vi "CSM Module Type.vi"(8 "Error in":errorcluster caption="error in (no error)", 11 "CSM Basic Refs":T2) -> (0 "error out":errorcluster, 2 "CSMType":T1, 3 "CSM Basic Refs (dup)":T2)   [LabVIEW 2017, in "CSM-Helper Utility.lvlib"]
doc: "### CSM Module Type.vi\n\n-- <b>Controls</b> --\n- <b>CSM Basic Refs</b>:\n\n-- <b>Indicators</b> --\n- <b>CSM Basic Refs (dup)</b>:"
uses:
  CSM-Helper Utility.lvlib
  CSM Basic Refs.ctl
  CSM Module Type.ctl
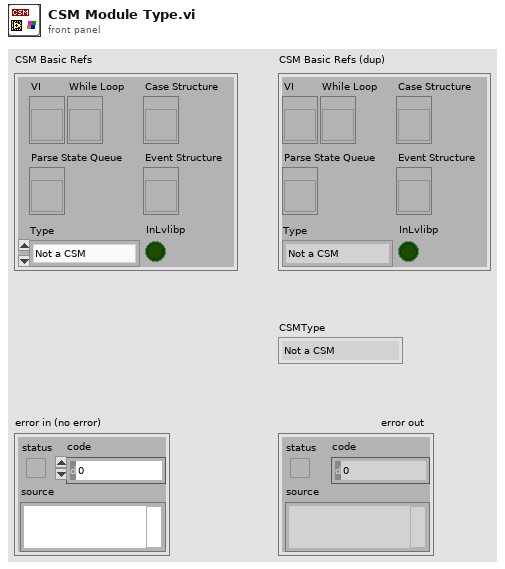
[diagram p1: front panel]
types:
  T1 = typedef "CSM-Helper Utility.lvlib/CSM Module Type.ctl" = enum16{"Not a CSM", "JKISM", "CSM"}
  T2 = typedef "CSM-Helper Utility.lvlib/CSM Basic Refs.ctl" = cluster{"VI":refnum<vi>, "While Loop":refnum<vi>, "Case Structure":refnum<vi>, "Parse State Queue":refnum<vi>, "Event Structure":refnum<vi>, "Type":T1, "InLvlibp":bool}
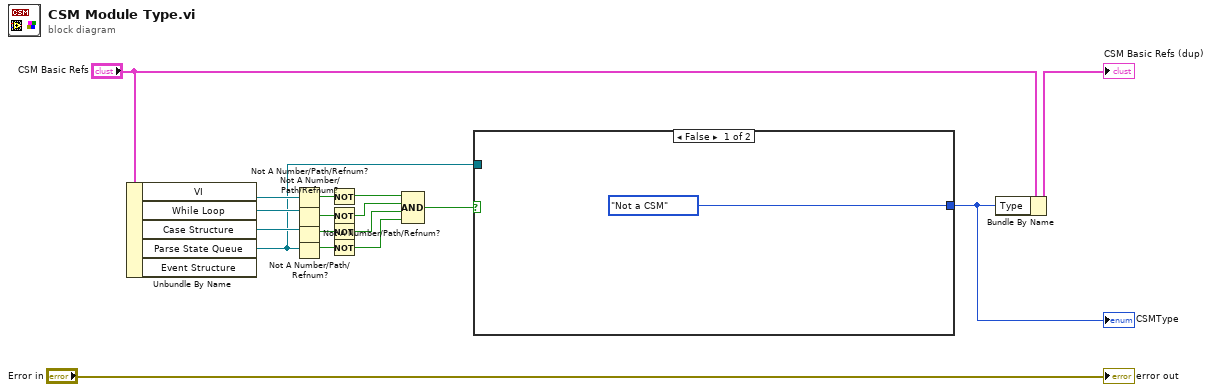
[diagram p0: block diagram]
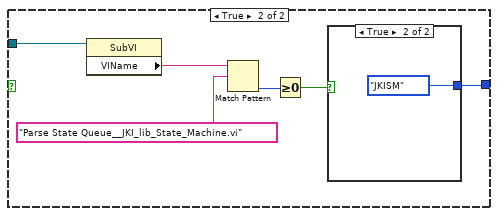
[diagram p2: hidden frame]
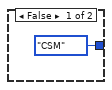
[diagram p3: hidden frame]
diagram:
  n1 = Unbundle By Name("CSM Basic Refs") -> ("VI"=w15:refnum<vi>, "While Loop"=w14:refnum<vi>, "Case Structure"=w12:refnum<vi>, "Parse State Queue"=w5:refnum<vi>)  [unwired: 1 out]
  n2 = Not A Number/Path/Refnum?(number/path/refnum=w15) -> (NaN/Path/Refnum?=w17:bool)
  n3 = Not A Number/Path/Refnum?(number/path/refnum=w14) -> (NaN/Path/Refnum?=w16:bool)
  n4 = Not A Number/Path/Refnum?(number/path/refnum=w12) -> (NaN/Path/Refnum?=w13:bool)
  n5 = Not A Number/Path/Refnum?(number/path/refnum=w5) -> (NaN/Path/Refnum?=w11:bool)
  n6 = Not(x=w17) -> (.not. x?=w10:bool)
  n7 = Not(x=w16) -> (.not. x?=w9:bool)
  n8 = Not(x=w13) -> (.not. x?=w8:bool)
  n9 = Not(x=w11) -> (.not. x?=w7:bool)
  n10 = Compound Arithmetic op=AND(w10, w9, w8, w7) -> (w6:bool)
  n11 = case shown="False" w6 {
    tunnel: [CSM_Module_Type."Not a CSM" w24] -> w1
    tunnel: w5 -> [_ w23]
    frame False {
    }
    frame True {
      n12 = property class="SubVI"(reference=w23) -> ("VIName"=w22:string)  [unwired: 1 in, 2 out]
      n13 = Match Pattern(string=w22, regular expression="Parse State Queue__JKI_lib_State_Machine.vi") -> (offset past match=w20:i32)  [unwired: 1 in, 3 out]
      n14 = Greater Or Equal To 0?(x=w20) -> (x >= 0?=w19:bool)
      n15 = case shown="True" w19 {
        tunnel: [CSM_Module_Type."CSM" CSM_Module_Type."JKISM"] -> w24
        frame False {
        }
        frame True {
        }
      }
    }
  }
  "CSMType" <- w1
  n16 = Bundle By Name(cluster="CSM Basic Refs", "Type"=w1) -> (→"CSM Basic Refs (dup)":T2)
  "error out" <- "Error in"
